vi "DeleteTemporaryPath.vi"(8 "error in (no error)":errorcluster, 11 "Folder_Mgmt":refnum<class "Folder_Mgmt.lvclass">) -> (0 "error out":errorcluster, 3 "Folder_Mgmt 2":refnum<class "Folder_Mgmt.lvclass">)   [LabVIEW 2016, in "Folder_Mgmt.lvclass"]
doc: "This VI deletes a DVR reference variable."
uses:
  Folder_Mgmt.lvclass
  Folder_Mgmt.lvclass/Folder_Mgmt.ctl
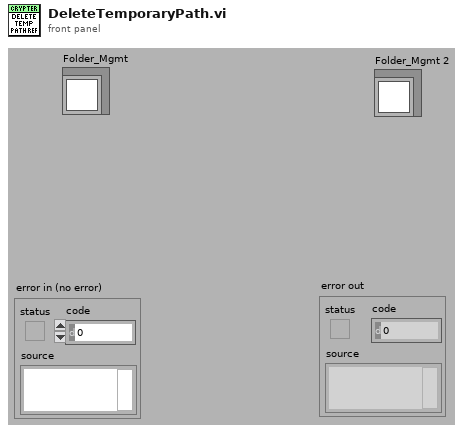
[diagram p1: front panel]
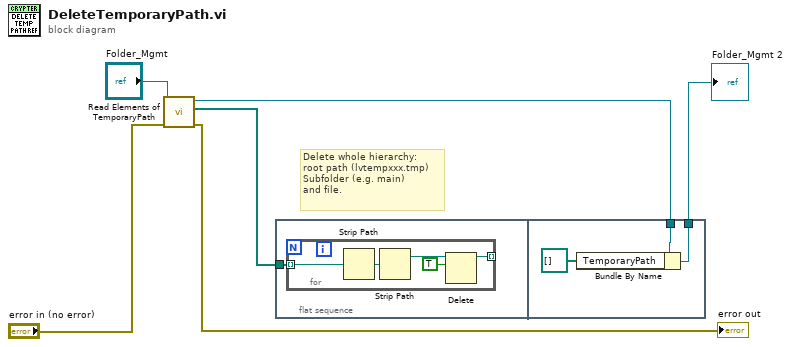
[diagram p0: block diagram]
diagram:
  # "Delete whole hierarchy:\nroot path (lvtempxxx.tmp)\nSubfolder (e.g. main)\nand file."
  n1 = call "Read Elements of TemporaryPath.vi"("error in (no error)"="error in (no error)", "Folder_Mgmt"="Folder_Mgmt") -> ("error out"=→"error out":errorcluster, "TemporaryPath"=w6:path[], "Folder_Mgmt 2"=w1:refnum<class "Folder_Mgmt.lvclass">)  [unwired: 7 in]
  n2 = flat-sequence {
    tunnel: w6 -> [w7]
    tunnel: w1 -> [w15]
    tunnel: [w13] -> w2
    frame #0 {
      n3 = for {
        tunnel: w7 -> [w12] mode=indexing
        tunnel: [w11] -> _ mode=indexing
        n4 = Strip Path(path=w12) -> (stripped path=w10:path)  [unwired: 1 out]
        n5 = Strip Path(path=w10) -> (stripped path=w9:path)  [unwired: 1 out]
        n6 = Delete(path (use dialog)=w9, entire hierarchy (F)=TRUE) -> (deleted path=w11:path)  [unwired: 3 in, 2 out]
      }
    }
    frame #1 {
      n7 = Bundle By Name(cluster=w15, "TemporaryPath"=path[] []) -> (w13:refnum<class "Folder_Mgmt.lvclass">)
    }
  }
  "Folder_Mgmt 2" <- w2
